vi "KVMap-Filter.vi"(8 "T->First/F->Second(F)":bool, 10 "filter":string, 11 "Cluster in":cluster{string[], string[]}) -> (3 "Cluster out":cluster{string[], string[]})   [LabVIEW 2014]
uses:
  <userlib>/_OpenG.lib/array/array.llb/Delete Elements from 1D Array (String)__ogtk.vi
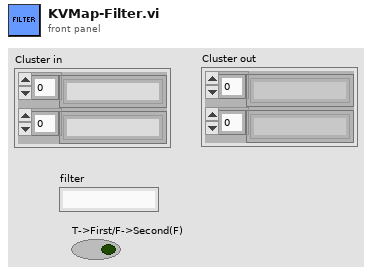
[diagram p1: front panel]
types:
  T1 = cluster{"array w/ subset deleted":string[], "array w/ subset deleted":string[]}
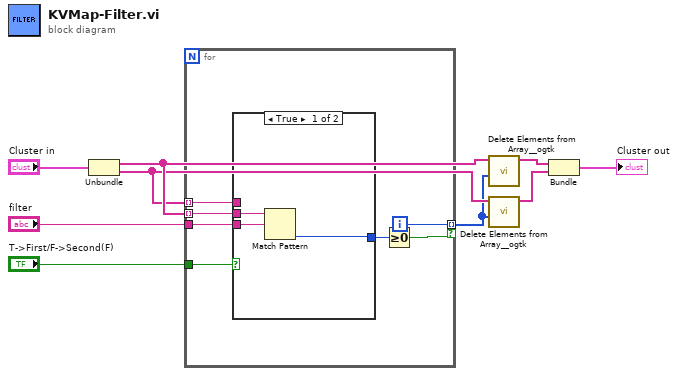
[diagram p0: block diagram]
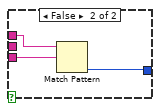
[diagram p2: hidden frame]
diagram:
  n1 = Unbundle("Cluster in") -> (w3:string[], w2:string[])
  n2 = for {
    tunnel: w2 -> [w16] mode=indexing
    tunnel: "T->First/F->Second(F)" -> [w15]
    tunnel: [w12] -> w1 mode=indexing if=w10
    tunnel: w3 -> [w14] mode=indexing
    tunnel: "filter" -> [w13]
    i -> [w12]
    n3 = case shown="True" w15 {
      tunnel: w13 -> [w19 w22]
      tunnel: w14 -> [w18 _]
      tunnel: w16 -> [_ w21]
      tunnel: [w17 w20] -> w11
      frame True {
        n4 = Match Pattern(string=w18, regular expression=w19) -> (offset past match=w17:i32)  [unwired: 1 in, 3 out]
      }
      frame False {
        n5 = Match Pattern(string=w21, regular expression=w22) -> (offset past match=w20:i32)  [unwired: 1 in, 3 out]
      }
    }
    n6 = Greater Or Equal To 0?(x=w11) -> (x >= 0?=w10:bool)
  }
  n7 = call-poly <userlib>:"Delete Elements from Array__ogtk.vi"("indices"=w1, "array"=w3) -> ("array w/ subset deleted"=w6:string[])  [unwired: 8 in, 1 out]
  n8 = call-poly <userlib>:"Delete Elements from Array__ogtk.vi"("indices"=w1, "array"=w2) -> ("array w/ subset deleted"=w7:string[])  [unwired: 8 in, 1 out]
  n9 = Bundle("array w/ subset deleted"=w6, "array w/ subset deleted"=w7) -> (→"Cluster out":T1)  [unwired: 1 in]
